vi "Sort HW.vi"(8 "error in (no error)":errorcluster, 11 "Hardware Settings in":refnum<class "Hardware Settings.lvclass">) -> (0 "error out":errorcluster, 1 "Saturation Hardware":refnum<class "Hardware Settings.lvclass">, 2 "Expansion Hardware":refnum<class "Hardware Settings.lvclass">)   [LabVIEW 2017, in "Hardware Settings.lvclass"]
uses:
  Hardware Settings.lvclass
  Hardware Settings.lvclass/Hardware Settings.ctl
  Hardware Types/Generic/Generic Hardware.lvclass/Generic Hardware.ctl
  Hardware Types/Generic/Accessors/Read Owning System.vi
  Accessors/Read Active Channels.vi
  Accessors/Write Active Channels.vi
  Hardware Types/Generic/Generic Hardware.lvclass
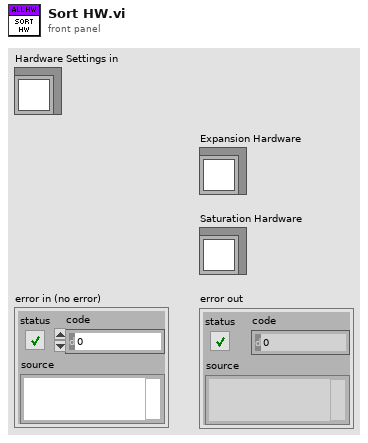
[diagram p1: front panel]
types:
  T1 = typedef "Generic Hardware.lvclass/Owning System.ctl" = enum16{"Saturation", "Expansion"}
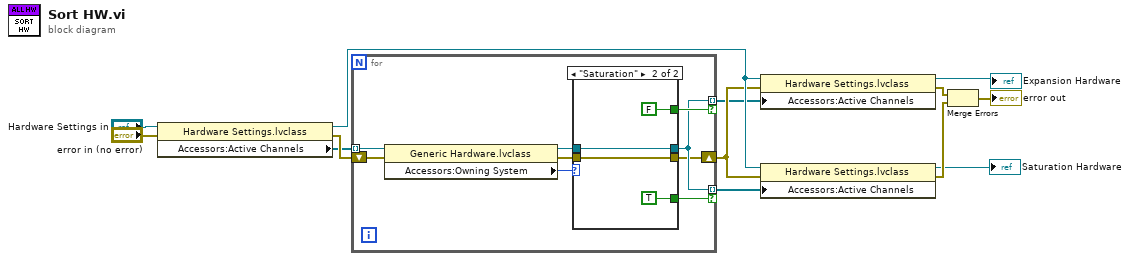
[diagram p0: block diagram]
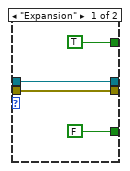
[diagram p2: hidden frame]
diagram:
  n1 = property class="Hardware Settings.lvclass"(reference="Hardware Settings in", error in="error in (no error)") -> (reference out=w13:refnum<class "Hardware Settings.lvclass">, error out=w8:errorcluster, "Accessors:Active Channels"=w3:refnum<class "Generic Hardware.lvclass">[])
  n2 = for {
    tunnel: w3 -> [w22] mode=indexing
    tunnel: [w18] -> w5 mode=indexing if=w19
    tunnel: [w18] -> w4 mode=indexing if=w17
    shift-right: [w14] -> w9
    shift-left: w8 -> [w16]
    n3 = property class="Generic Hardware.lvclass"(reference=w22, error in=w16) -> (reference out=w20:refnum<class "Generic Hardware.lvclass">, error out=w15:errorcluster, "Accessors:Owning System"=w21:T1)
    n4 = case shown="\"Saturation\"" w21 {
      tunnel: w20 -> [w26 w30]
      tunnel: [w26 w30] -> w18
      tunnel: [TRUE FALSE] -> w19
      tunnel: [FALSE TRUE] -> w17
      tunnel: w15 -> [w23 w27]
      tunnel: [w23 w27] -> w14
      frame "Expansion" {
      }
      frame "Saturation" {
      }
    }
  }
  n5 = property class="Hardware Settings.lvclass"(reference=w13, error in=w9, "Accessors:Active Channels"=w5) -> (reference out=→"Expansion Hardware":refnum<class "Hardware Settings.lvclass">, error out=w10:errorcluster)
  n6 = property class="Hardware Settings.lvclass"(reference=w13, error in=w9, "Accessors:Active Channels"=w4) -> (reference out=→"Saturation Hardware":refnum<class "Hardware Settings.lvclass">, error out=w12:errorcluster)
  n7 = Merge Errors(w10, w12) -> (→"error out":errorcluster)
